vi "Read SPX.vi"(8 "error in (no error)":errorcluster, 11 "All Albums":T1) -> (0 "error out":errorcluster, 3 "All Albums":T1)   [LabVIEW 2015]
uses:
  Controls & Type Defs/AlbumArray.ctl
  <vilib>/regexp/Match Regular Expression.xnode
panel:
  out "Raw Text From File":string
  # "(For debugging)"
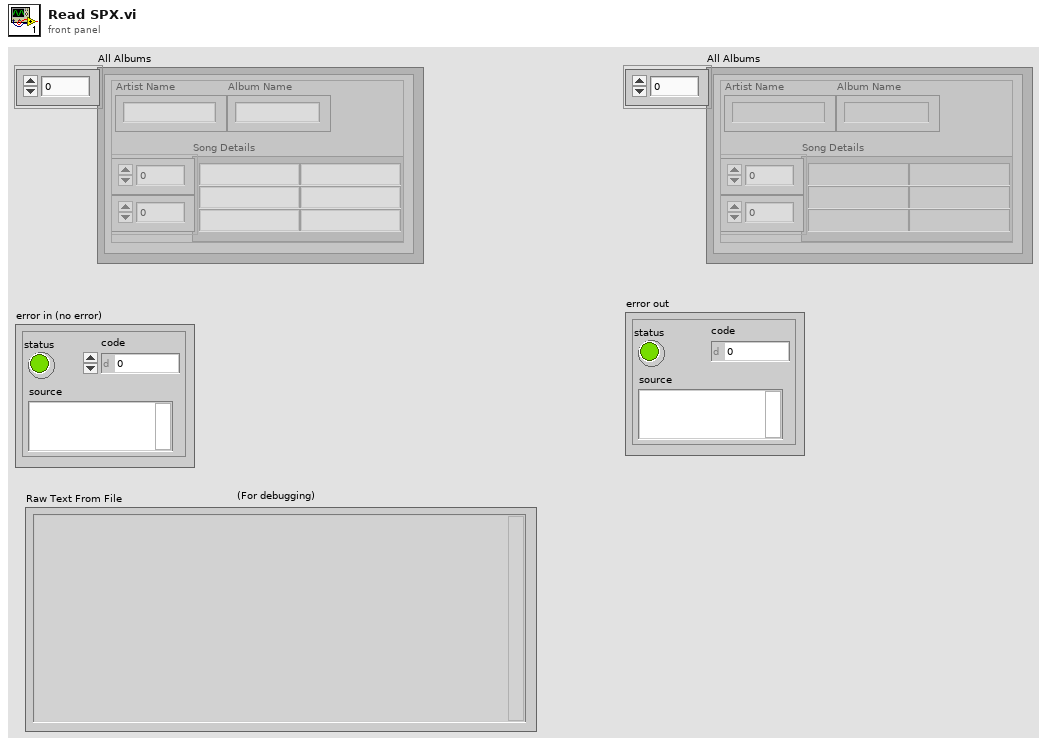
[diagram p1: front panel]
types:
  T1 = typedef "AlbumArray.ctl" = cluster{"Artist Name":string, "Album Name":string, "Song Details":string[][]}[]
  T2 = cluster{"Artist Name":string, "Album Name":string, "Song Details":string[][]}
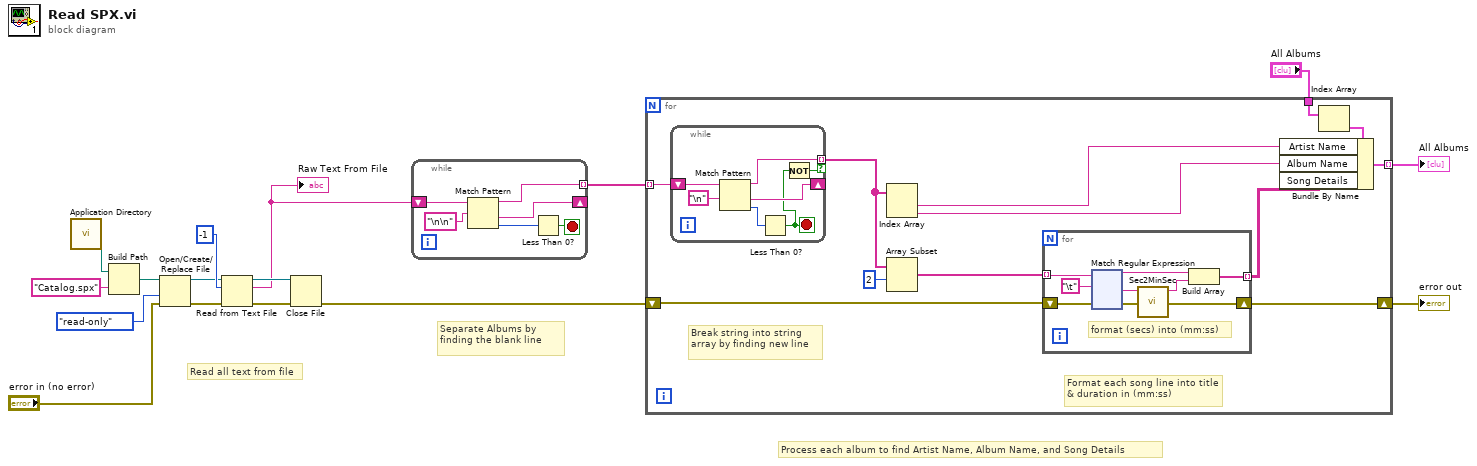
[diagram p0: block diagram]
diagram:
  # "Read all text from file"
  # "Process each album to find Artist Name, Album Name, and Song Details"
  # "Separate Albums by finding the blank line"
  n1 = call <vilib>:"Application Directory.vi"() -> ("Application Directory"=w7:path)
  n2 = Build Path(base path=w7, name or relative path="Catalog.spx") -> (appended path=w9:path)
  n3 = Open/Create/Replace File(file path (use dialog)=w9, error in="error in (no error)", access (0:read/write)=enum16{"read/write", "read-only", "write-only"}."read-only") -> (refnum out=w12:refnum<file>, error out=w13:errorcluster)  [unwired: 3 in, 1 out]
  n4 = Read from Text File(file (use dialog)=w12, count=-1, error in=w13) -> (refnum out=w15:refnum<file>, text=w5:string, error out=w16:errorcluster)  [unwired: 1 in, 1 out]
  "Raw Text From File" <- w5
  n5 = Close File(refnum=w15, error in=w16) -> (error out=w3:errorcluster)  [unwired: 1 out]
  n6 = while {
    shift-right: [w18] -> _
    shift-left: w5 -> [w22]
    tunnel: [w17] -> w6 mode=indexing
    stop <- w19 stop-if-true
    n7 = Match Pattern(string=w22, regular expression="\n\n") -> (before substring=w17:string, after substring=w18:string, offset past match=w20:i32)  [unwired: 1 in, 1 out]
    n8 = Less Than 0?(x=w20) -> (x < 0?=w19:bool)
  }
  n9 = for {
    tunnel: w6 -> [w32] mode=indexing
    tunnel: [w28] -> w1 mode=indexing
    shift-right: [w27] -> w4
    shift-left: w3 -> [w26]
    tunnel: "All Albums" -> [w25]
    # "Format each song line into title & duration in (mm:ss)"
    # "Break string into string array by finding new line"
    n10 = while {
      shift-right: [w161] -> _
      shift-left: w32 -> [w162]
      tunnel: [w160] -> w34 mode=indexing if=w158
      stop <- w157 stop-if-true
      n11 = Match Pattern(string=w162, regular expression="\n") -> (before substring=w160:string, after substring=w161:string, offset past match=w163:i32)  [unwired: 1 in, 1 out]
      n12 = Less Than 0?(x=w163) -> (x < 0?=w157:bool)
      n13 = Not(x=w157) -> (.not. x?=w158:bool)
    }
    n14 = Index Array "Index Array"(array=w34) -> (element #1=w30:string, element #2=w29:string)  [unwired: 2 in]
    n15 = Array Subset "Array Subset"(array=w34, index=2) -> (w31:string[])  [unwired: 1 in]
    n16 = for {
      tunnel: w31 -> [w42] mode=indexing
      tunnel: [w39] -> w23 mode=indexing
      shift-right: [w36] -> w27
      shift-left: w26 -> [w35]
      # "format (secs) into (mm:ss)"
      n17 = xnode "Match Regular Expression"("input string"=w42, "regular expression"="\t", "error in"=w35) -> ("before match"=w41:string, "after match"=w38:string, "error out"=w36:errorcluster)  [unwired: 3 in, 2 out]
      n18 = call "Sec2MinSec.vi"("duration (s)"=w38) -> ("duration (mm:ss)"=w37:string)  [unwired: 10 in]
      n19 = Build Array(w41, w37) -> (w39:string[])
    }
    n20 = Index Array(array=w25) -> (element=w24:T2)  [unwired: 1 in]
    n21 = Bundle By Name(cluster=w24, "Artist Name"=w30, "Album Name"=w29, "Song Details"=w23) -> (w28:T2)
  }
  "error out" <- w4
  "All Albums" <- w1
